vi "read oos.vi"() -> ()   [LabVIEW 2012]
panel:
  in  "stop":bool
  out "progress":i32(slide)=3096 scale=0.0..45806.0
  out "front pic":T1(plugin-control)
  in  "file":path
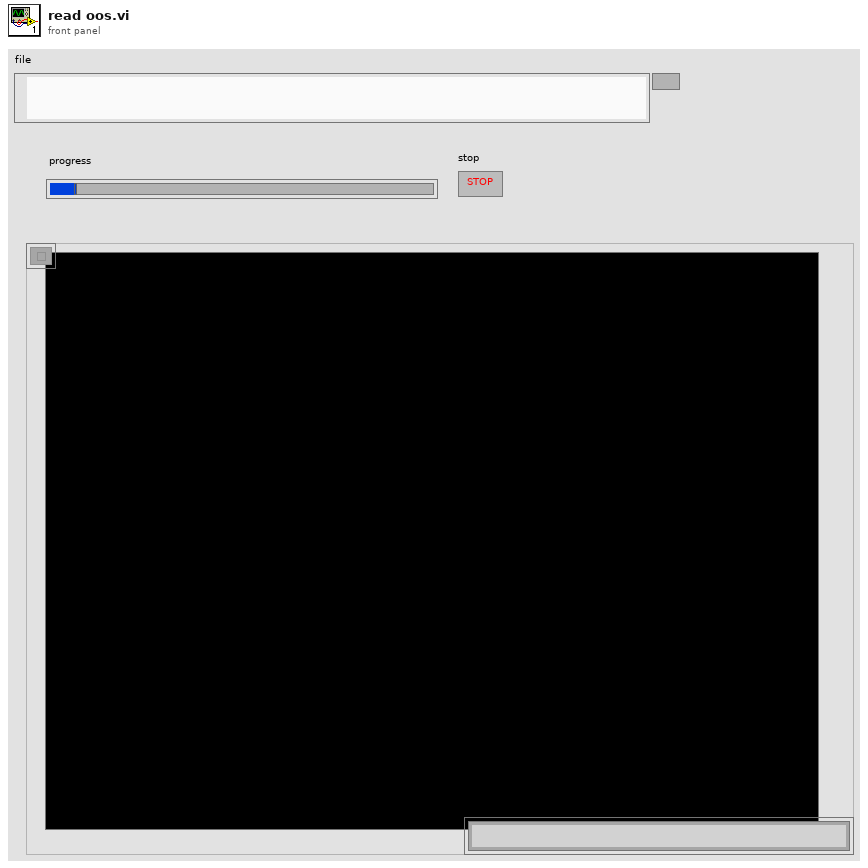
[diagram p1: front panel]
types:
  T1 = typedef "IMAQ Image.ctl" = refnum<image>
  T2 = typedef "Image Type" = u32
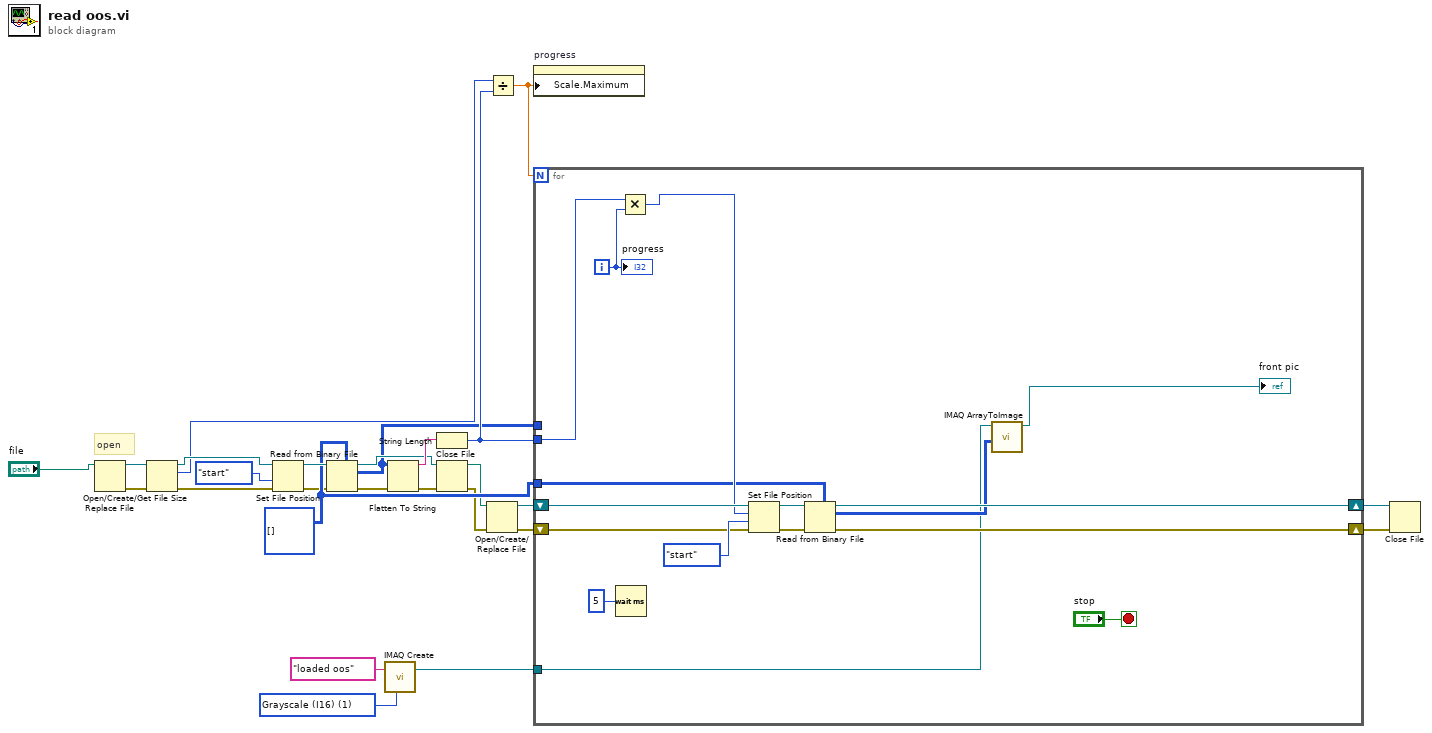
[diagram p0: block diagram]
diagram:
  w5 = T2 1 items=["Grayscale (U8)", "Grayscale (I16)", "Grayscale (SGL)", "Complex (CSG)", "RGB (U32)", "HSL (U32)", "RGB (U64)", "Grayscale (U16)"] ("Image Type")
  w15 = i16[][] [] ("Image Pixels (I16)")
  # "open"
  n1 = Open/Create/Replace File(file path (use dialog)="file") -> (refnum out=w26:refnum<file>, error out=w25:errorcluster)  [unwired: 5 in, 1 out]
  n2 = Get File Size(file=w26, error in=w25) -> (refnum out=w23:refnum<file>, size (in bytes)=w19:i64, 0:w13:errorcluster)
  n3 = Set File Position(refnum=w23, from (0:start)=enum16{"start", "end", "current"}."start", error in=w13) -> (refnum out=w22:refnum<file>, error out=w12:errorcluster)  [unwired: 1 in]
  n4 = Read from Binary File(5:w15, 8:w12, 11:w22) -> (0:w20:errorcluster, 2:w9:i16[][], 3:w17:refnum<file>)  [unwired: 3 in, 1 out]
  n5 = call "IMAQ Create"("Image Name"="loaded oos", "Image Type"=w5) -> ("New Image"=w6:T1)  [unwired: 3 in, 1 out]
  n6 = Flatten To String(anything=w9, error in (no error)=w20) -> (data string=w21:string, error out=w11:errorcluster)  [unwired: 2 in, 1 out]
  n7 = String Length(string=w21) -> (length=w16:i32)
  n8 = Close File(refnum=w17, error in=w11) -> (path=w3:path, error out=w2:errorcluster)
  n9 = Open/Create/Replace File(file path (use dialog)=w3, error in=w2) -> (refnum out=w4:refnum<file>, error out=w1:errorcluster)  [unwired: 4 in, 1 out]
  n10 = Divide(x=w19, y=w16) -> (x/y=w18:dbl)
  n11 = property on="progress" class="Slide (strict)"("Scale.Maximum"=w18) -> ()  [unwired: 2 in, 2 out]
  n12 = for {
    N: w18 -> [_]
    shift-right: [w31] -> w14
    shift-left: w4 -> [w41]
    tunnel: w16 -> [w40]
    tunnel: w15 -> [w34]
    shift-right: [w32] -> w10
    shift-left: w1 -> [w36]
    tunnel: w9 -> [_]
    tunnel: w6 -> [w29]
    i -> [w33]
    stop <- "stop" stop-if-true
    n13 = Wait (ms)(milliseconds to wait=u32 5) -> ()  [unwired: 1 out]
    n14 = Multiply(x=w40, y=w33) -> (x*y=w39:i32)
    n15 = Set File Position(offset (in bytes) (0)=w39, refnum=w41, from (0:start)=enum16{"start", "end", "current"}."start", error in=w36) -> (refnum out=w37:refnum<file>, error out=w38:errorcluster)
    n16 = Read from Binary File(5:w34, 8:w38, 11:w37) -> (0:w32:errorcluster, 2:w30:i16[][], 3:w31:refnum<file>)  [unwired: 3 in, 1 out]
    n17 = call "IMAQ ArrayToImage"("Image Pixels (I16)"=w30, "Image"=w29) -> ("Image Out"=→"front pic":T1)  [unwired: 8 in, 1 out]
    "progress" <- w33
  }
  n18 = Close File(refnum=w14, error in=w10) -> ()  [unwired: 2 out]
